vi "PH_Switch.set GUI Refs.vi"(0 "VI in":refnum<vi>, 2 "GUI Refs":T1, 5 "error in (no error)":errorcluster) -> (14 "VI out":refnum<vi>, 19 "error out":errorcluster)   [LabVIEW 2014, in "PH_Switch.lvlib"]
uses:
  PH_Switch.lvlib
  PH_Switch.GUI Refs.ctl
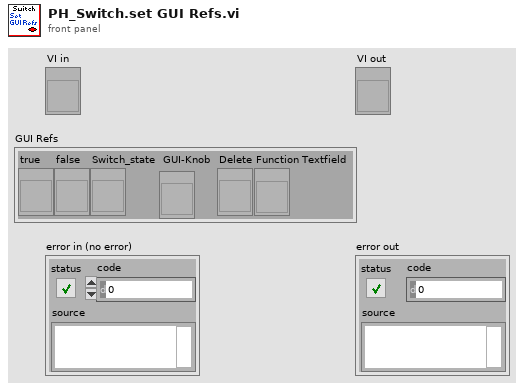
[diagram p1: front panel]
types:
  T1 = typedef "PH_Switch.lvlib/PH_Switch.GUI Refs.ctl" = cluster{"true":refnum<vi>, "false":refnum<vi>, "Switch_state":refnum<vi>, "GUI-Knob":refnum<vi>, "Delete":refnum<vi>, "Function Textfield":refnum<vi>}
  T2 = typedef "PH_Switch.lvlib/PH_Switch.i attribute.ctl" = cluster{"GUI Refs":T1, "Status true":T3, "Status false":T3, "Status Switch State":T3, "remote controlled":bool, "Tagname":cluster{"Switch":string, "True":string, "False":string}, "Beckhoff Instance":string, "Caption":cluster{"True":string, "False":string}, "Default State":string}
  T3 = typedef "PH_StatusHandler.lvlib/PH_StatusHandler.Status.ctl" = i16
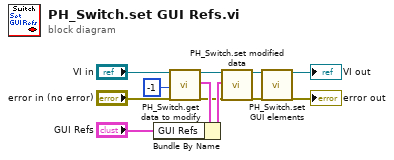
[diagram p0: block diagram]
diagram:
  n1 = call "PH_Switch.get data to modify.vi"("i ref in"="VI in", "ms timeout (10000)"=-1, "error in (no error)"="error in (no error)") -> ("i ref out"=w5:refnum<vi>, "i attribute"=w10:T2, "error out"=w6:errorcluster)  [unwired: 13 in, 1 out]
  n2 = Bundle By Name(cluster=w10, "GUI Refs"="GUI Refs") -> (w11:T2)
  n3 = call "PH_Switch.set modified data.vi"("i ref in"=w5, "i attribute"=w11, "error in (no error)"=w6) -> ("i ref out"=w3:refnum<vi>, "error out"=w4:errorcluster)  [unwired: 15 in]
  n4 = call "PH_Switch.set GUI elements.vi"("i ref in"=w3, "error in (no error)"=w4) -> ("i ref out"=→"VI out":refnum<vi>, "error out"=→"error out":errorcluster)  [unwired: 16 in]
